vi "Low rep rate beam pointing correction from kHz images.vi"() -> ()   [LabVIEW 2020]
doc: "The Parallel Processing (Optimized Performance) example shows how to process multiple images in parallel when using a ring acquisition. Images acquired from a camera are stored in a ring buffer and references to each image are pushed to a queue. Each worker loop removes a reference from the queue and processes the image.\n\nIn this example, image processing is simulated by a time delay that can be adjusted while the VI is running. When processing is complete, <B>IMAQdx Release Image</B> must be called in order to free space in the ring buffer."
uses:
  <vilib>/vision/Image Controls.llb/IMAQ Image.ctl
  <vilib>/vision/driver/IMAQdx.llb/IMAQdx Acquisition Mode.ctl
  <vilib>/vision/driver/IMAQdx.llb/IMAQdx Buffer Number Mode.ctl
  <vilib>/vision/driver/NI_Vision_Acquisition_Software.lvlib
  <resource>/objmgr/imaqdx.rc
panel:
  out "processed in burst":u32
  out "error IO":errorcluster
  out "remaining elements":T2(array[cluster])
  out "# elements in queue":i32
  out "error out":errorcluster
  out "loop time":u32
  out "Waveform Chart":T3(graph)
  out "Image":T1(plugin-control)
  in  "threshold fraction":sgl=0.8
  in  "Use threshold fraction":bool=TRUE
  out "Images Behind":u32
  in  "Range":cluster{"Lower value":sgl, "Upper value":sgl}={"Lower value"=128.0, "Upper value"=255.0} caption="Threshold Range" {"Upper value" format="%.2f"; "Lower value" format="%.2f"}
  out "Lost Buffer Count":u32
  in  "# Images in Burst":i32=200
  out "Images in Queue":i32
  out "Images Processed":u32
  out "Current Buffer Number":u32
  in  "Camera Name":refnum<k21> caption="IMAQdx Session"
  in  "Stop":bool
  # "Overview: Processes multiple extracted images in parallel when using a ring acquisition.\nRequirements: Vision Acquisition Software\nInstructions:\n1. Select the Camera Name\n2. Run the VI"
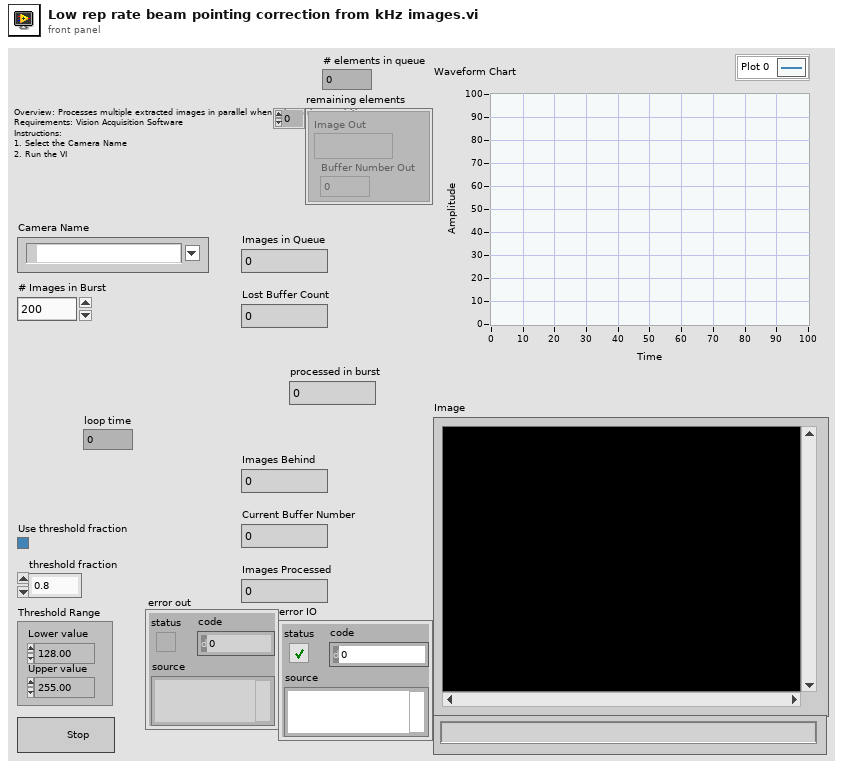
[diagram p1: front panel]
types:
  T1 = typedef "IMAQ Image.ctl" = refnum<image>
  T2 = cluster{"Image Out":T1, "Buffer Number Out":u32}[]
  T3 = cluster{"X Centroid":sgl, "Y Centroid":sgl, "X Centroid":sgl, "Y Centroid":sgl}
  T4 = typedef "IMAQdx.ctl" = refnum<k21>
  T5 = typedef "NI_Vision_Acquisition_Software.lvlib/IMAQdx Acquisition Mode.ctl" = enum32{"One Shot", "Continuous"}
  T6 = typedef "NI_Vision_Acquisition_Software.lvlib/IMAQdx Buffer Number Mode.ctl" = enum32{"Next", "Last", "Buffer Number", "Every", "Last New"}
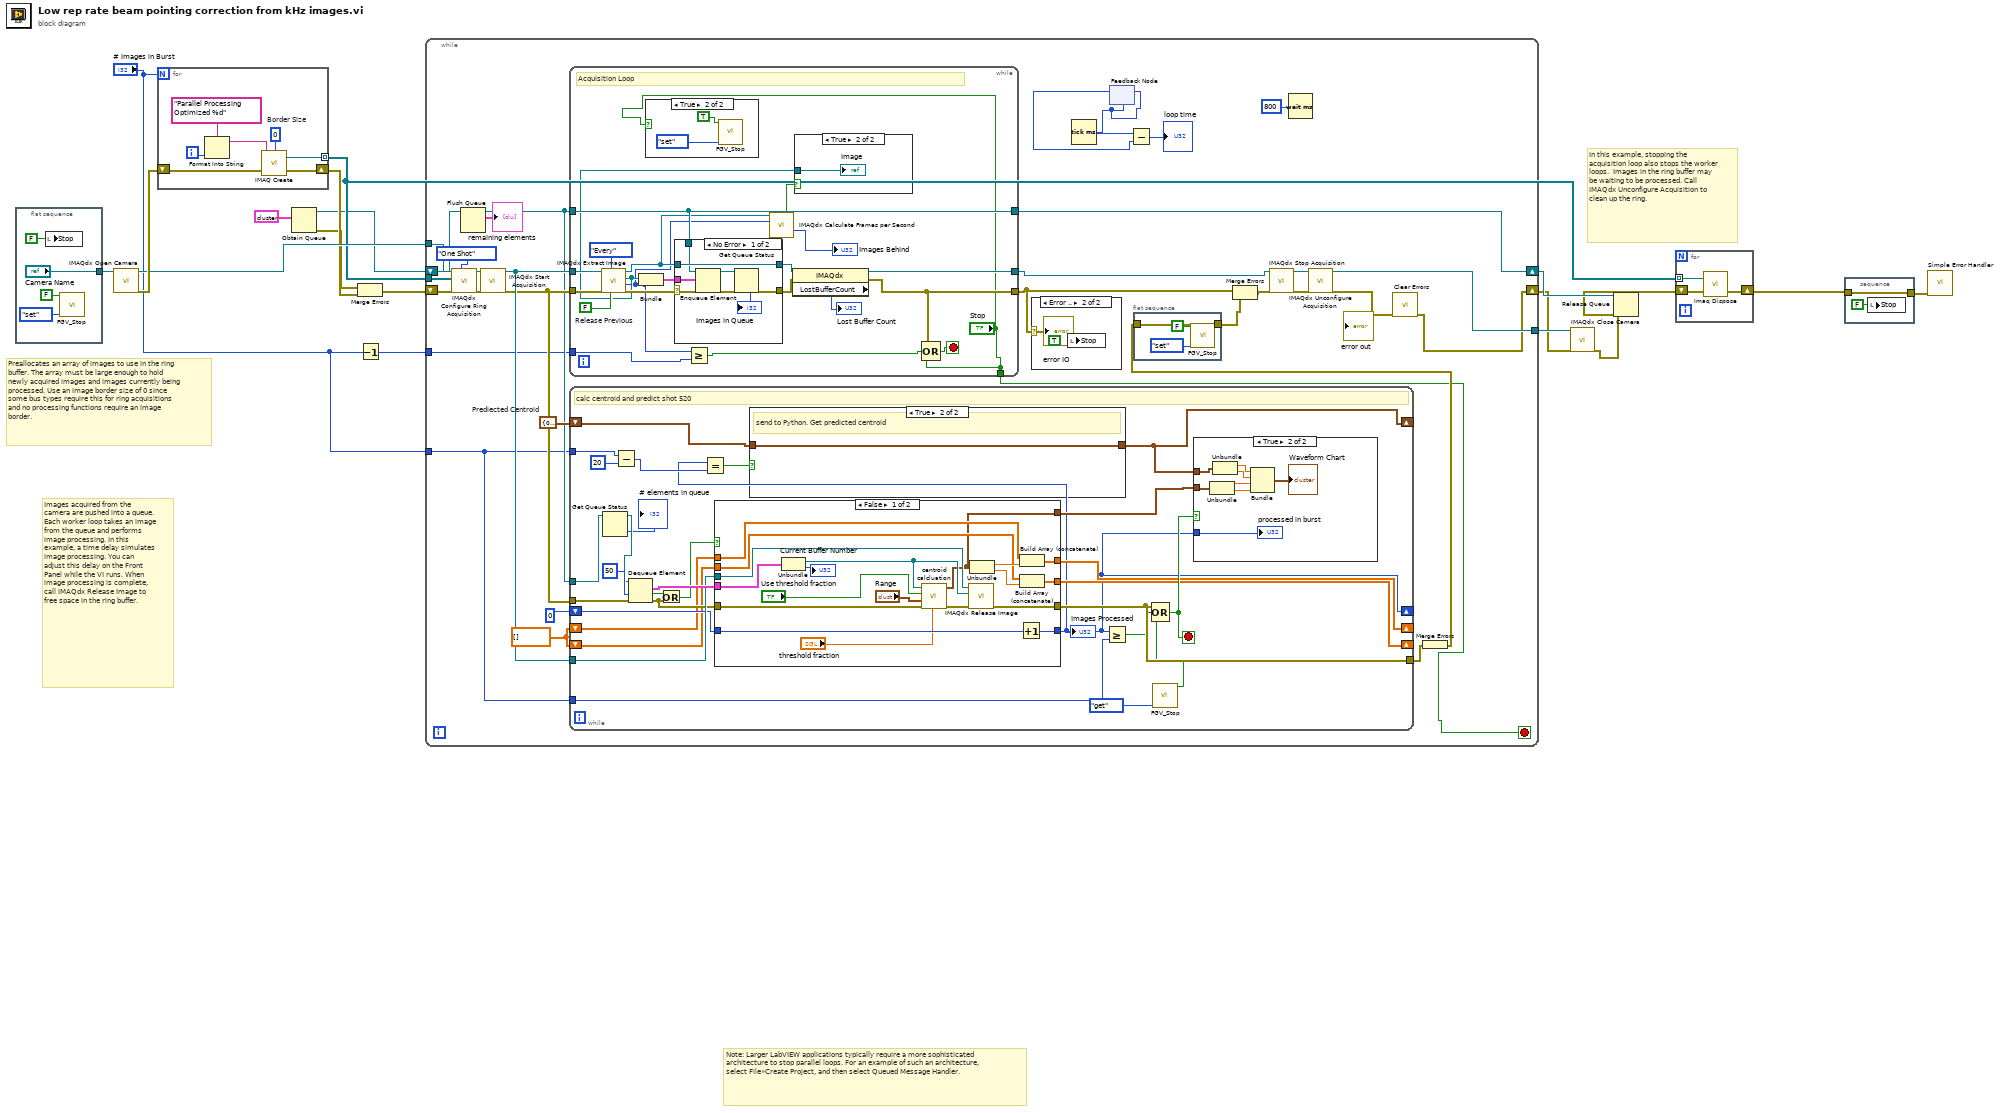
[diagram p0: block diagram]
diagram:
  # "In this example, stopping the acquisition loop also stops the worker loops.  Images in the ring buffer may be waiting to be processed. Call IMAQdx Unconfigure Acquisition to clean up the ring."
  # "Images acquired from the camera are pushed into a queue. Each worker loop takes an image from the queue and performs image processing. In this example, a time delay simulates image processing. You can adjust this delay on the Front Panel while the VI runs. When image processing is complete, call IMAQdx Release Image to free space in the ring buffer."
  # "Preallocates an array of images to use in the ring buffer. The array must be large enough to hold newly acquired images and images currently being processed. Use an image border size of 0 since some bus types require this for ring acquisitions and no processing functions require an image border."
  # "Note: Larger LabVIEW applications typically require a more sophisticated architecture to stop parallel loops. For an example of such an architecture, select File»Create Project, and then select Queued Message Handler."
  n1 = flat-sequence {
    tunnel: ["Camera Name"] -> w16
    frame #0 {
      n2 = local write "Stop"(FALSE ("Stop")) -> ()
      n3 = call "FGV_Stop.vi"("command"=enum16{"set", "get"}."set", "stop"=FALSE) -> ()  [unwired: 9 in, 1 out]
    }
  }
  n4 = call <vilib>:"IMAQdx Open Camera.vi"("Session In"=w16) -> ("error out"=w15:errorcluster, "Session Out"=w14:T4)  [unwired: 2 in, 7 out]
  n5 = for {
    N: "# Images in Burst" -> [_]
    tunnel: [w28] -> w8 mode=indexing
    shift-right: [w27] -> w11
    shift-left: w15 -> [w29]
    i -> [w26]
    w23 = 0  # Border Size
    n6 = Format Into String(format string="Parallel Processing Optimized %d" ("Image Name"), w26) -> (resulting string=w25:string)  [unwired: 2 in, 1 out]
    n7 = call "IMAQ Create"("Border Size"=w23, "Image Name"=w25, "error in (no error)"=w29) -> ("New Image"=w28:T1, "error out"=w27:errorcluster)  [unwired: 1 in, 1 out]
  }
  n8 = Obtain Queue(element data type=cluster{"Image Out":T1, "Buffer Number Out":u32} {"Image Out"=refnum, "Buffer Number Out"=0}) -> (queue out=w6:refnum<queue>, error out=w10:errorcluster)  [unwired: 4 in, 1 out]
  n9 = Merge Errors(w10, w11) -> (w12:errorcluster)
  n10 = Decrement(x="# Images in Burst") -> (x-1=w2:i32)
  n11 = while {
    tunnel: w14 -> [w62]
    tunnel: w8 -> [w59]
    shift-right: [w33] -> w3
    shift-left: w12 -> [w61]
    shift-right: [w60] -> w9
    shift-left: w6 -> [w58]
    tunnel: [w34] -> w5
    tunnel: w2 -> [w31]
    tunnel: "# Images in Burst" -> [w30]
    stop <- w35 stop-if-true
    w43 = cluster{"X Centroid":sgl, "Y Centroid":sgl} {"X Centroid"=0.0, "Y Centroid"=0.0}  # Prediected Centroid
    w44 = sgl[] []
    n12 = call <vilib>:"IMAQdx Configure Ring Acquisition.vi"("Mode"=IMAQdx_Acquisition_Mode."One Shot" ("Continuous?"), "error in"=w61, "Images"=w59, "Session In"=w62) -> ("error out"=w54:errorcluster, "Session Out"=w55:T4)  [unwired: 5 in, 1 out]
    n13 = Flush Queue(queue=w58) -> (queue out=w37:refnum<queue>, remaining elements=→"remaining elements":T2)  [unwired: 1 in, 1 out]
    n14 = call <vilib>:"IMAQdx Start Acquisition.vi"("error in"=w54, "Session In"=w55) -> ("error out"=w49:errorcluster, "Session Out"=w50:T4)  [unwired: 8 out]
    n15 = while {
      tunnel: w49 -> [w150]
      tunnel: w50 -> [w147]
      tunnel: w37 -> [w140]
      tunnel: [w146] -> w51
      tunnel: [w144] -> w32
      tunnel: [w140] -> w60
      tunnel: ["Stop"] -> w35
      tunnel: w31 -> [w131]
      stop <- w132 stop-if-true
      w148 = FALSE  # Release Previous
      # "Acquisition Loop"
      n16 = call <vilib>:"IMAQdx Extract Image.vi"("Release Previous (true)"=w148, "Buffer Number Mode (Next)"=IMAQdx_Buffer_Number_Mode."Every" ("Buffer Number Mode"), "error in"=w150, "Session In"=w147) -> ("error out"=w143:errorcluster, "Buffer Number Out"=w134:u32, "Image Out"=w135:T1, "Session Out"=w137:T4)  [unwired: 4 in]
      n17 = Bundle("Image Out"=w135, "Buffer Number Out"=w134) -> (w141:cluster{"Image Out":T1, "Buffer Number Out":u32})  [unwired: 1 in]
      n18 = case shown="True" "Stop" {
        frame False {
        }
        frame True {
          n19 = call "FGV_Stop.vi"("command"=enum16{"set", "get"}."set", "stop"=TRUE) -> ()  [unwired: 9 in, 1 out]
        }
      }
      n20 = case shown="No Error" w143 {
        selector: w143 -> [w157 w162]
        tunnel: [w158 w163] -> w142
        tunnel: w137 -> [w158 w163]
        tunnel: w141 -> [w156 _]
        tunnel: w140 -> [w155 _]
        tunnel: [w154 w162] -> w139
        frame No Error {
          n21 = Enqueue Element(queue=w155, element=w156, error in (no error)=w157) -> (queue out=w160:refnum<queue>, error out=w161:errorcluster)  [unwired: 1 in, 1 out]
          n22 = Get Queue Status(queue=w160, error in (no error)=w161) -> (error out=w154:errorcluster, # elements in queue=→"Images in Queue":i32)  [unwired: 1 in, 6 out]
        }
        frame Error {
        }
      }
      n23 = Greater Or Equal?(x=w134, y=w131) -> (x >= y?=w133:bool)
      n24 = call <vilib>:"IMAQdx Calculate Frames per Second.vi"("Session In"=w137, "Buffer Number"=w134) -> ("Update Display"=w136:bool, "Images Behind"=→"Images Behind":i32)  [unwired: 7 in, 5 out]
      n25 = property class="IMAQdx"(reference=w142, error in=w139) -> (reference out=w146:T4, error out=w144:errorcluster, "LostBufferCount"=→"Lost Buffer Count":u32)
      n26 = case shown="True" w136 {
        tunnel: w135 -> [_ w153]
        frame False {
        }
        frame True {
          "Image" <- w153
        }
      }
      n27 = Compound Arithmetic op=OR(w144, w133, "Stop") -> (w132:bool)
    }
    n28 = while {
      tunnel: [w84] -> w45
      tunnel: w37 -> [w76]
      tunnel: w50 -> [w91]
      shift-right: [w66] -> _
      shift-left: u32 0 -> [w90]
      tunnel: w49 -> [w89]
      shift-right: [w82] -> _
      shift-left: w44 -> [w83]
      shift-right: [w81] -> _
      shift-left: w44 -> [w80]
      shift-right: [w78] -> _
      shift-left: w43 -> [w79]
      tunnel: w30 -> [w73]
      tunnel: w30 -> [w69]
      stop <- w85 stop-if-true
      # "calc centroid and predict shot 520"
      n29 = Get Queue Status(queue=w76) -> (queue out=w75:refnum<queue>, # elements in queue=→"# elements in queue":i32)  [unwired: 2 in, 6 out]
      n30 = Subtract(x=w73, y=20) -> (x-y=w71:i32)
      n31 = Dequeue Element(queue=w75, timeout in ms (-1)=50 ("timeout in ms"), error in (no error)=w89) -> (element=w92:cluster{"Image Out":T1, "Buffer Number Out":u32}, timed out?=w87:bool, error out=w86:errorcluster)  [unwired: 1 out]
      n32 = Or(x=w87, y=w86) -> (x .or. y?=w88:bool)
      n33 = case shown="False" w88 {
        tunnel: w86 -> [w116 w126]
        tunnel: w92 -> [w122 _]
        tunnel: [w121 w126] -> w84
        tunnel: w91 -> [w120 _]
        tunnel: w90 -> [w118 w125]
        tunnel: [w117 w125] -> w66
        tunnel: w83 -> [w110 w124]
        tunnel: [w108 w124] -> w82
        tunnel: [w106 w123] -> w81
        tunnel: w80 -> [w105 w123]
        tunnel: [w104 _] -> w77
        frame False {
          n34 = Unbundle(w122) -> ("Image Out"=w113:T1, "Buffer Number Out"=→"Current Buffer Number":u32)
          n35 = call "centroid calcluation.vi"("threshold fraction"="threshold fraction", "error in (no error)"=w116, "Range"="Range", "Use threshold fraction"="Use threshold fraction", "Refnum in"=w113) -> ("error out"=w115:errorcluster, "Centroid"=w104:cluster{"X Centroid":sgl, "Y Centroid":sgl})  [unwired: 4 in, 1 out]
          n36 = call <vilib>:"IMAQdx Release Image.vi"("error in"=w115, "Image"=w113, "Session In"=w120) -> ("error out"=w121:errorcluster)  [unwired: 7 in, 1 out]
          n37 = Unbundle(w104) -> ("X Centroid"=w109:sgl, "Y Centroid"=w107:sgl)
          n38 = Increment(x=w118) -> (x+1=w117:u32)
          n39 = Build Array (concatenate)(w110, w109) -> (w108:sgl[])
          n40 = Build Array (concatenate)(w105, w107) -> (w106:sgl[])
        }
        frame True {
          # "Empty queue or error.\nNothing to process."
        }
      }
      "Images Processed" <- w66
      n41 = Equal?(x=w66, y=w71) -> (x = y?=w65:bool)
      n42 = case shown="True" w65 {
        tunnel: w79 -> [w94 w95]
        tunnel: [w94 w95] -> w78
        frame False {
        }
        frame True {
          # "send to Python. Get predicted centroid"
        }
      }
      n43 = Greater Or Equal?(x=w66, y=w69) -> (x >= y?=w70:bool)
      n44 = call "FGV_Stop.vi"("command"=enum16{"set", "get"}."get") -> ("stop"=w67:bool)  [unwired: 10 in]
      n45 = Compound Arithmetic op=OR(w84, w70, w67) -> (w85:bool)
      n46 = case shown="True" w85 {
        tunnel: w78 -> [_ w102]
        tunnel: w77 -> [_ w103]
        tunnel: w66 -> [_ w96]
        frame False {
        }
        frame True {
          n47 = Unbundle(w103) -> ("X Centroid"=w99:sgl, "Y Centroid"=w98:sgl)
          n48 = Unbundle(w102) -> ("X Centroid"=w101:sgl, "Y Centroid"=w100:sgl)
          n49 = Bundle("X Centroid"=w101, "Y Centroid"=w100, "X Centroid"=w99, "Y Centroid"=w98) -> (→"Waveform Chart":T3)  [unwired: 1 in]
          "processed in burst" <- w96
        }
      }
    }
    n50 = case shown="Error .." w32 {
      selector: w32 -> [_ w63]
      frame No Error {
      }
      frame Error {
        n51 = local write "Stop"(TRUE ("Stop")) -> ()
        "error IO" <- w63
      }
    }
    n52 = Tick Count (ms)() -> (millisecond timer value=w42:u32)
    n53 = feedback #1(w42) -> (w41:u32)
    n54 = feedback-in #1(w42) -> ()
    n55 = Subtract(x=w42, y=w41) -> (x-y=→"loop time":u32)
    n56 = flat-sequence {
      tunnel: w48 -> [w127]
      tunnel: [w127] -> w47
      frame #0 {
        n57 = call "FGV_Stop.vi"("command"=enum16{"set", "get"}."set", "stop"=FALSE) -> ()  [unwired: 9 in, 1 out]
      }
    }
    n58 = Merge Errors(w32, w47) -> (w52:errorcluster)
    n59 = call <vilib>:"IMAQdx Stop Acquisition.vi"("error in"=w52, "Session In"=w51) -> ("error out"=w56:errorcluster, "Session Out"=w57:T4)  [unwired: 8 out]
    n60 = Wait (ms)(milliseconds to wait=u32 800) -> ()  [unwired: 1 out]
    n61 = call <vilib>:"IMAQdx Unconfigure Acquisition.vi"("error in"=w56, "Session In"=w57) -> ("error out"=w39:errorcluster, "Session Out"=w34:T4)  [unwired: 8 out]
    "error out" <- w39
    n62 = call <vilib>:"Clear Errors.vi"("error in (no error)"=w39) -> ("error out"=w33:errorcluster)  [unwired: 5 in, 1 out]
    n63 = Merge Errors(w45) -> (w48:errorcluster)
  }
  n64 = call <vilib>:"IMAQdx Close Camera.vi"("error in"=w3, "Session In"=w5) -> ("error out"=w4:errorcluster)  [unwired: 9 out]
  n65 = Release Queue(queue=w9, error in (no error)=w4) -> (error out=w7:errorcluster)  [unwired: 1 in, 2 out]
  n66 = for {
    shift-right: [w165] -> w17
    shift-left: w7 -> [w166]
    tunnel: w8 -> [w164] mode=indexing
    n67 = call "Imaq Dispose"("Image"=w164, "error in (no error)"=w166) -> ("error out"=w165:errorcluster)  [unwired: 4 in]
  }
  n68 = stacked-sequence {
    tunnel: [w167] -> w18
    tunnel: w17 -> [w167]
    frame #0 {
      n69 = local write "Stop"(FALSE ("Stop")) -> ()
    }
  }
  n70 = call <vilib>:"Simple Error Handler.vi"("error in (no error)"=w18) -> ()  [unwired: 4 in, 5 out]
